vi "Read Word.vi"(11 "GDSII.DataType.Word in":refnum<class "GDSII.DataType.Word.lvclass">) -> (2 "Word":i16[](array[numeric]), 3 "GDSII.DataType.Word out":refnum<class "GDSII.DataType.Word.lvclass">)   [LabVIEW 2019, in "GDSII.DataType.Word.lvclass"]
uses:
  GDSII.DataType.Word.lvclass
  GDSII.DataType.Word.lvclass/GDSII.DataType.Word.ctl
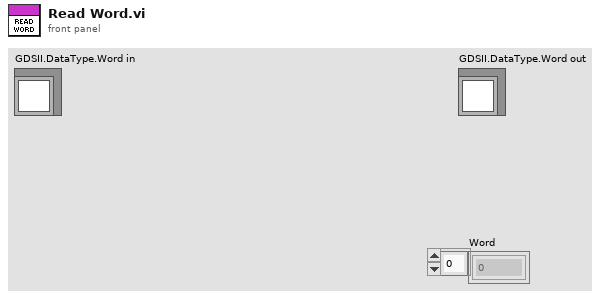
[diagram p1: front panel]
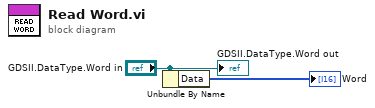
[diagram p0: block diagram]
diagram:
  n1 = Unbundle By Name("GDSII.DataType.Word in") -> ("Data"=→"Word":i16[])
  "GDSII.DataType.Word out" <- "GDSII.DataType.Word in"
